vi "Stop Core.vi"(10 "final error code":i32, 11 "WS Test Client in":refnum<class "WS Test Client.lvclass">) -> (3 "WS Test Client out":refnum<class "WS Test Client.lvclass">)   [LabVIEW 2016, in "WS Full LabVIEW Test.lvlib" / "WS Test Client.lvclass"]
doc: "In addition to the following, this method also sends a message to the monitor to notify it that the actor has stopped execution.\n\n(<B>Filename</B>: Actor Framework.lvlib:Actor.lvclass:Stop Core.vi)\n\nDefines what the actor does before it stops. Use the <B>final error code</B> input to determine whether the actor shut down in response to an error.\n\nBy default, this method does nothing. A descendant class may override it to define behavior, such as shutting down any processes the actor initiated in its override of the Actor Core method.\n\nCopyright: MGI\n\nAuthored by Derek Trepanier\nsupport@mooregoodideas.com\nwww.mooregoodideas.com\n\nCopyright (c) 2014, Moore Good Ideas, Inc.\n\nAll rights reserved.\n\nRedistribution and use in source and binary forms, with or without modification, are permitted provided that the following conditions are met:\n\n * Redistributions of source code must retain the above copyright notice, this list of conditions and the following disclaimer.\n * Redistributions in binary form must reproduce the above copyright notice, this list of conditions and the following disclaimer in the documentation and/or other materials provided with the distribution.\n * Neither the name of Moore Good Ideas, Inc. nor the names of its contributors may be used to endorse or promote products derived from this software without specific prior written permission.\n\nTHIS SOFTWARE IS PROVIDED BY THE COPYRIGHT HOLDERS AND CONTRIBUTORS \"AS IS\" AND ANY EXPRESS OR IMPLIED WARRANTIES, INCLUDING, BUT NOT LIMITED TO, THE IMPLIED WARRANTIES OF MERCHANTABILITY AND FITNESS FOR A PARTICULAR PURPOSE ARE DISCLAIMED. IN NO EVENT SHALL THE COPYRIGHT OWNER OR CONTRIBUTORS BE LIABLE FOR ANY DIRECT, INDIRECT, INCIDENTAL, SPECIAL, EXEMPLARY, OR CONSEQUENTIAL DAMAGES (INCLUDING, BUT NOT LIMITED TO, PROCUREMENT OF SUBSTITUTE GOODS OR SERVICES; LOSS OF USE, DATA, OR PROFITS; OR BUSINESS INTERRUPTION) HOWEVER CAUSED AND ON ANY THEORY OF LIABILITY, WHETHER IN CONTRACT, STRICT LIABILITY, OR TORT (INCLUDING NEGLIGENCE OR OTHERWISE) ARISING IN ANY WAY OUT OF THE USE OF THIS SOFTWARE, EVEN IF ADVISED OF THE POSSIBILITY OF SUCH DAMAGE."
uses:
  WS Test Client.lvclass
  WS Test Client.lvclass/WS Test Client.ctl
  <vilib>/MGI/Monitored Actor/Monitored Actor/Monitored Actor/Monitored Actor.lvclass
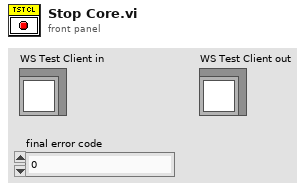
[diagram p1: front panel]
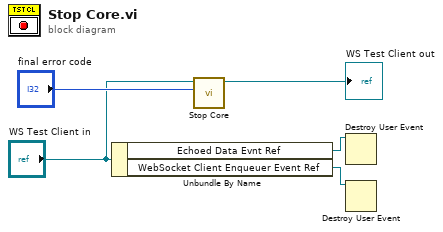
[diagram p0: block diagram]
diagram:
  n1 = Unbundle By Name("WS Test Client in") -> ("Echoed Data Evnt Ref"=w2:refnum<user-event>, "WebSocket Client Enqueuer Event Ref"=w1:refnum<user-event>)
  n2 = call-parent "Stop Core.vi"("final error code"="final error code", "Monitored Actor in"="WS Test Client in") -> ("Monitored Actor out"=→"WS Test Client out":refnum<class "WS Test Client.lvclass">)  [unwired: 9 in]
  n3 = Destroy User Event(user event=w2) -> ()  [unwired: 1 in, 1 out]
  n4 = Destroy User Event(user event=w1) -> ()  [unwired: 1 in, 1 out]
